vi "Subview Template.vi"(8 "error in (no error)":errorcluster, 10 "Subview Stop Event":refnum<user-event>, 11 "Subsystem URL":refnum<k21>) -> ()   [LabVIEW 2024]
doc: "The template for creating a subview."
uses:
  Shared/User Event - Stop.lvlib
panel:
  out "error out":errorcluster
  in  "Stop":bool
  # "This is a subview template. You can duplicate this template to create your own subview.\n\nComplete the following steps to create your own subview:\n    1. Duplicate this subview. \n    2. Insert a switch button on the left of the Detailed View, add an event handler in the event handling loop to send out a new message standing for the created subview.\n    3. Create a corresponding message handler in the Message Handling Loop in the Detailed View. You can append the message to the current \"Alarm & Event List\", \"Historical Trend\", \"Subsystem View\" case.\n    4. Add the switch button reference in the \"Initialize\" case.\n    5. Add the static VI reference of the created subview in the Open Subview VI Reference.vi. \n    6. Run and test your subview in the Detailed View.\n\nNote:\n    * Set the subview VI to preallocated clone reentrant execution, because several copies of the subview may exist simultaneously.\n    * Save the front panel with an appropriate size to fit the subpanel size of the Detailed View."
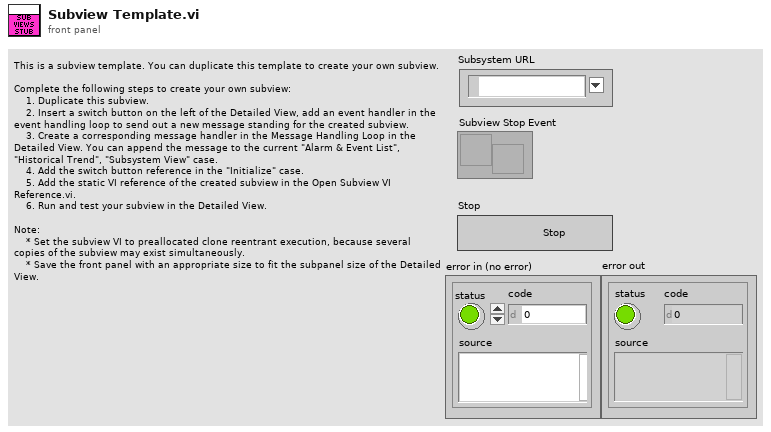
[diagram p1: front panel]
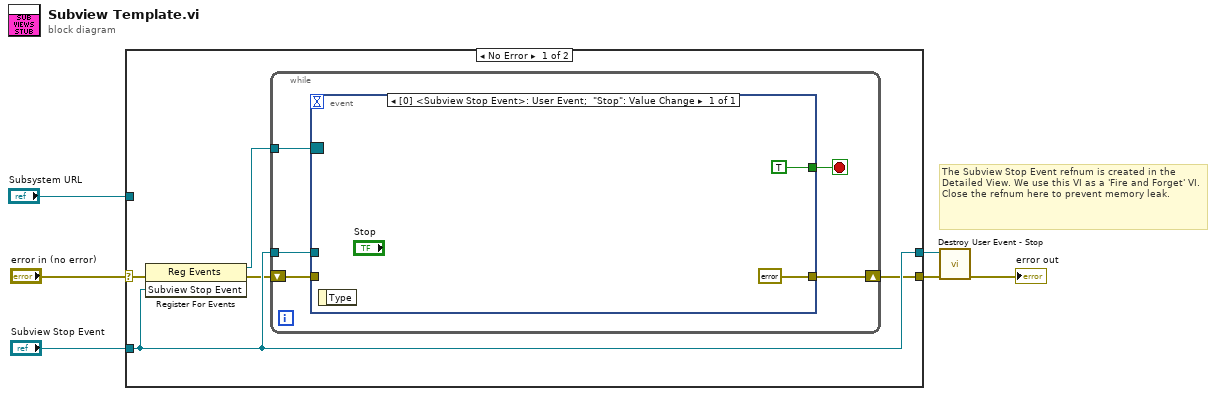
[diagram p0: block diagram]
diagram:
  # "The Subview Stop Event refnum is created in the Detailed View. We use this VI as a 'Fire and Forget' VI. Close the refnum here to prevent memory leak."
  n1 = case shown="No Error" "error in (no error)" {
    selector: "error in (no error)" -> [w7 w19]
    tunnel: "Subview Stop Event" -> [w11 w20]
    tunnel: [w10 w19] -> w3
    tunnel: [w11 w20] -> w4
    tunnel: "Subsystem URL" -> [_ _]
    frame No Error {
      n2 = register-events(error in=w7, w11) -> (reference out=w9:refnum<event-registration>, error out=w8:errorcluster)  [unwired: 1 in]
      n3 = while {
        shift-right: [w13] -> w10
        shift-left: w8 -> [w14]
        tunnel: w9 -> [w15]
        tunnel: w11 -> [w12]
        stop <- w16 stop-if-true
        n4 = event shown="[0] <Subview Stop Event>: User Event;  \"Stop\": Value Change" {
          selector: w15 -> [_]
          dyn-events: _ -> [_]
          timeout: _ -> [_]
          tunnel: [TRUE] -> w16
          tunnel: w14 -> [_]
          tunnel: [errorcluster {"status"=FALSE, "code"=0, "source"=""} ("error out")] -> w13
          tunnel: w12 -> [_]
          event User Event; "Stop": Value Change {
            n5 = event-data() -> ()  [unwired: 1 in, 1 out]
          }
        }
      }
    }
    frame Error {
    }
  }
  n6 = call "Destroy User Event - Stop.vi"("error in (no error)"=w3, "User Event - Stop"=w4) -> ("error out"=→"error out":errorcluster)  [unwired: 9 in]
